vi "hydraharp_receive_buffer.vi"(8 "error in (no error)":errorcluster, 11 "hydraharp in":refnum<class "hydraharp.lvclass">) -> (0 "error out":errorcluster, 1 "stop":bool, 2 "queue_timed_out":bool, 3 "hydraharp out":refnum<class "hydraharp.lvclass">)   [LabVIEW 2015, in "hydraharp.lvclass"]
uses:
  hydraharp.lvclass
  hydraharp.lvclass/hydraharp.ctl
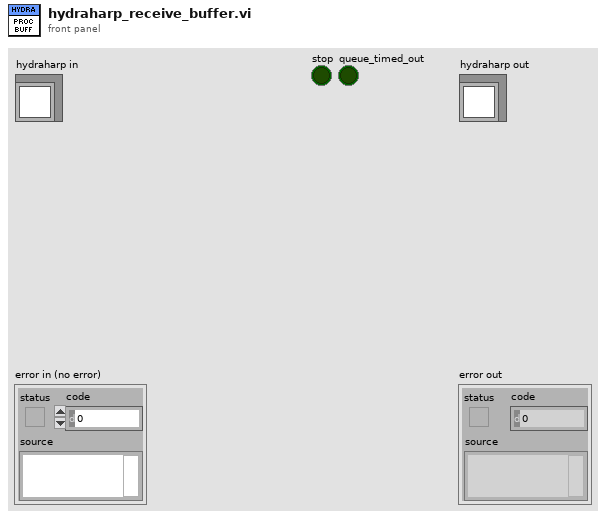
[diagram p1: front panel]
types:
  T1 = typedef "hpanel_acq_modes.ctl" = u16
  T2 = typedef "hydraharp_fifo_queue_data.ctl" = cluster{"fifo_buffer":u32[], "fifo_action":T3}
  T3 = typedef "hydraharp_fifo_actions.ctl" = enum16{"stop", "new_data"}
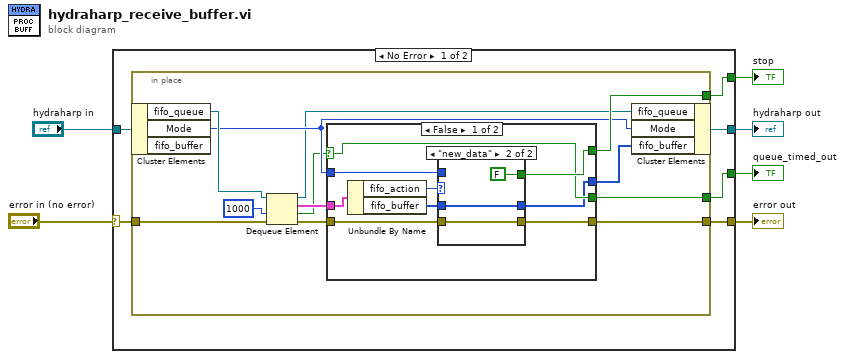
[diagram p0: block diagram]
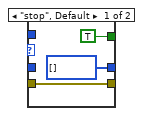
[diagram p2: hidden frame]
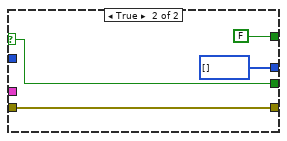
[diagram p3: hidden frame]
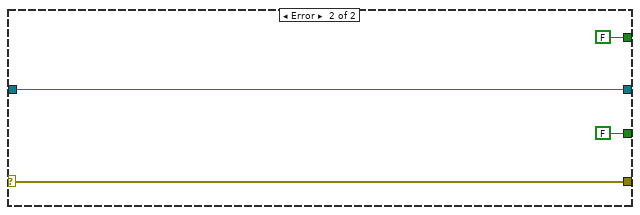
[diagram p4: hidden frame]
diagram:
  n1 = case shown="No Error" "error in (no error)" {
    selector: "error in (no error)" -> [w11 w47]
    tunnel: [w9 w47] -> w5
    tunnel: [w8 w46] -> w3
    tunnel: "hydraharp in" -> [w12 w46]
    tunnel: [w10 FALSE] -> w2
    tunnel: [w7 FALSE] -> w1
    frame No Error {
      n2 = in-place {
        in-place-border: w11 -> [w22]
        in-place-border: [w20] -> w10
        in-place-border: [w18] -> w9
        in-place-border: [w14] -> w7
        n3 = in-place-cluster #1(w12) -> ("fifo_queue"=w24:refnum<queue>, "Mode"=w17:T1)  [unwired: 1 out]
        n4 = Dequeue Element(queue=w24, timeout in ms (-1)=1000, error in (no error)=w22) -> (queue out=w16:refnum<queue>, element=w21:T2, timed out?=w15:bool, error out=w19:errorcluster)
        n5 = case shown="False" w15 {
          selector: w15 -> [w26 w41]
          tunnel: w21 -> [w33 _]
          tunnel: [w31 FALSE] -> w20
          tunnel: w19 -> [w29 w43]
          tunnel: [w28 w43] -> w18
          tunnel: w17 -> [w27 _]
          tunnel: [w26 w41] -> w14
          tunnel: [w25 u32[] [] ("fifo_buffer")] -> w13
          frame False {
            n6 = Unbundle By Name(w33) -> ("fifo_action"=w32:T3, "fifo_buffer"=w30:u32[])
            n7 = case shown="\"new_data\"" w32 {
              tunnel: [TRUE FALSE] -> w31
              tunnel: w30 -> [_ w37]
              tunnel: w27 -> [_ _]
              tunnel: w29 -> [w35 w38]
              tunnel: [w35 w38] -> w28
              tunnel: [u32[] [] ("fifo_buffer") w37] -> w25
              frame "stop", Default {
              }
              frame "new_data" {
              }
            }
          }
          frame True {
          }
        }
        n8 = in-place-cluster #1("fifo_queue"=w16, "Mode"=w17, "fifo_buffer"=w13) -> (w8:refnum<class "hydraharp.lvclass">)
      }
    }
    frame Error {
    }
  }
  "error out" <- w5
  "hydraharp out" <- w3
  "stop" <- w2
  "queue_timed_out" <- w1
